vi "Alternative Get MSG Queue.vi"(8 "error in":errorcluster, 11 "SEQ in":refnum<class "SEQ.lvclass">) -> (0 "error out":errorcluster, 2 "seqMsg":string[](array[string])=["1:09:27 PM\tValve to oxygen changed to TRUE.", "1:09:27 PM\tO2 flow set to 500.000000.", "1:09:32 PM\tMax orifice flow recorded.   Flow was 248.806366.", "1:09:42 PM\tStandard wait time elapsed.", "1:09:54 PM\tStandard wait time elapsed.", "1:09:55 PM\tLaser RMS stable in every cell. RSE Values: 0.000000\t0.000000\r\n", "1:09:55 PM\tSpeaker position changed to TRUE.", "1:09:55 PM\tO2 flow set to 248.806366.", "1:10:01 PM\tOzone stable in every cell.  Begin collecting data. RSE Values: 0.043430\t0.043108\t0.043108\t0.043537\t0.043537\t0.047428\t0.047428\t0.043882\t0.043882\t0.044978\t0.044978\t0.043616\t0.043616\t0.042956\r\n", "1:10:21 PM\tCollection step complete.", "1:10:21 PM\tO2 flow set to 186.604774.", "1:10:27 PM\tOzone stable in every cell.  Begin collecting data. RSE Values: 0.049616\t0.048562\t0.048562\t0.048143\t0.048143\t0.048496\t0.048678\t0.048678\t0.047656\t0.047656\t0.046716\t0.046716\t0.046716\r\n", "1:10:47 PM\tCollection step complete.", "1:10:47 PM\tO2 flow set to 124.403183.", "1:10:53 PM\tOzone stable in every cell.  Begin collecting data. RSE Values: 0.045074\t0.045269\t0.045269\t0.045371\t0.045371\t0.046657\t0.046657\t0.044803\t0.044803\t0.046626\t0.046626\t0.044248\t0.044248\t0.044248\r\n", "1:11:13 PM\tCollection step complete.", "1:11:13 PM\tO2 flow set to 62.201591.", "1:11:19 PM\tOzone stable in every cell.  Begin collecting data. RSE Values: 0.047075\t0.046939\t0.046939\t0.049594\t0.049594\t0.046739\t0.046655\t0.046655\t0.046655\t0.048990\t0.048989\t0.048989\t0.048989\r\n", "1:11:39 PM\tCollection step complete.", "1:11:39 PM\tData displayed!", "1:11:39 PM\tSpeaker position changed to FALSE.", "1:11:39 PM\tValve to oxygen changed to FALSE.", "1:11:39 PM\tO2 flow set to 0.000000.", "1:11:49 PM\tStandard wait time elapsed.", "1:12:02 PM\tStandard wait time elapsed."] caption="Messages")   [LabVIEW 2012, in "Sequence Composition.lvlib" / "SEQ.lvclass"]
doc: "Retrieve messages from the message queue. Since this calls a message reference, there is no need to wait for the response."
uses:
  SEQ.lvclass
  SEQ.lvclass/SEQ.ctl
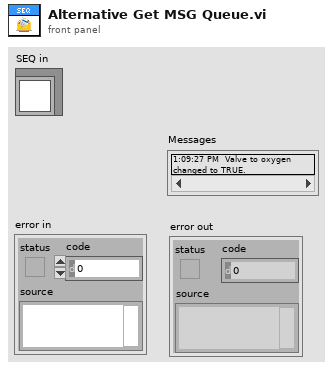
[diagram p1: front panel]
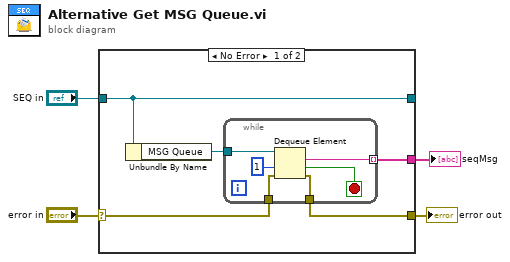
[diagram p0: block diagram]
diagram:
  n1 = case shown="No Error" "error in" {
    selector: "error in" -> [w7 w17]
    tunnel: [w6 w17] -> w3
    tunnel: [w9 w16] -> _
    tunnel: "SEQ in" -> [w9 w16]
    tunnel: [w5 _] -> w1
    frame No Error {
      n2 = Unbundle By Name(w9) -> ("MSG Queue"=w8:refnum<queue>)
      n3 = while {
        tunnel: w8 -> [w15]
        tunnel: [w12] -> w5 mode=indexing
        tunnel: w7 -> [w11]
        tunnel: [w10] -> w6
        stop <- w13 stop-if-true
        n4 = Dequeue Element(queue=w15, timeout in ms (-1)=1, error in (no error)=w11) -> (element=w12:string, timed out?=w13:bool, error out=w10:errorcluster)  [unwired: 1 out]
      }
    }
    frame Error {
    }
  }
  "error out" <- w3
  "seqMsg" <- w1
